vi "Scan.vi"() -> ()   [LabVIEW 2017, in "HP4192A IA.lvclass"]
uses:
  HP4192A IA.lvclass
  Global/GPIB Numbers.vi
  <vilib>/Utility/file.llb/Write To Spreadsheet File (DBL).vi
  File IO/File IO.lvclass
panel:
  in  "Number of Averages":u16 max=20 step=1
  in  "Averaging?":bool
  in  "Frequencies":string
  out "Measurements vs. Frequency":cluster{"Y":dbl[], "Y":dbl[]}[](graph)=[{"Y"=[5.0, 5.0, 5.0, 5.0, 5.0], "Y"=[-246999.99999999997, -1063000.0, -361000.0, -401000.0, -539000.0]}]
  in  "Delay between\nsteps":u32=500
  in  "?":bool
  in  "Append?":bool
  out "Current Frequency":dbl
  in  "?":bool
  in  "L":bool
  in  "C":bool
  in  "R":bool
  in  "Z":bool
  in  "Output File":path=path "C:/Data/Dielectric Measurements/2013 Measurements/.csv"
  # "Measure"
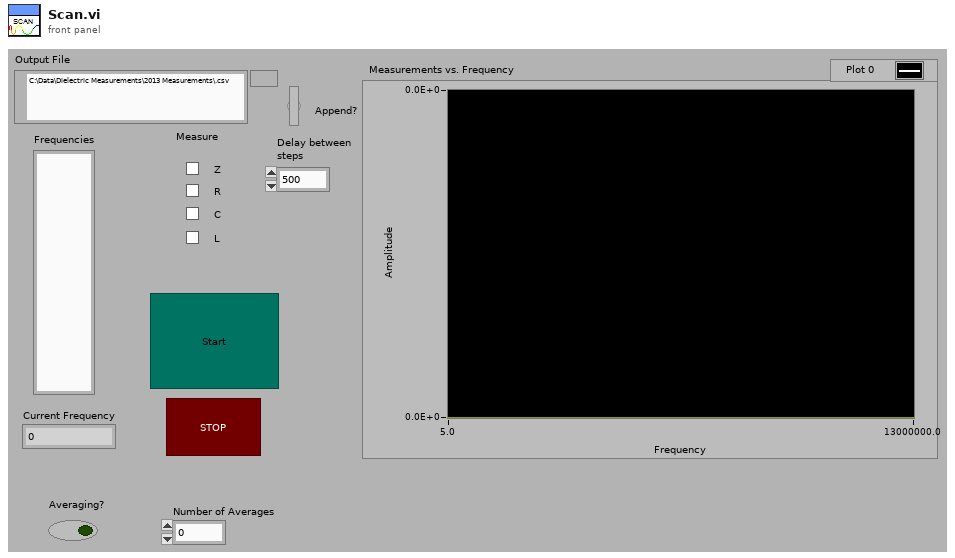
[diagram p1: front panel]
types:
  T1 = typedef "GPIB Type Def.ctl" = cluster{"Name":string, "bus":dbl, "GPIB":dbl, "GPIB as string":string, "byte":i32, "VISA Resource Name":refnum<visa-resource-name>}
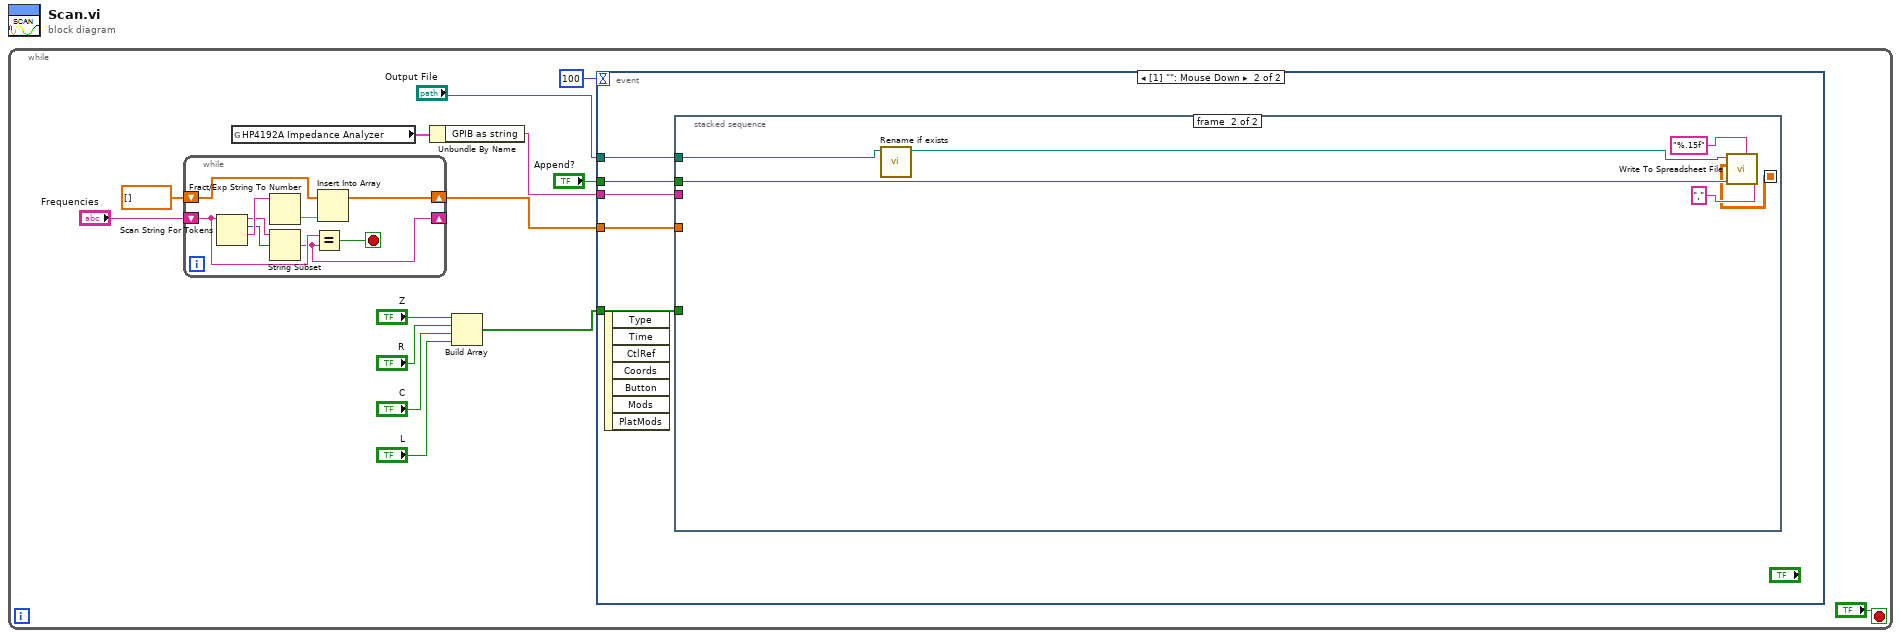
[diagram p0: block diagram]
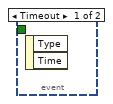
[diagram p2: hidden frame]
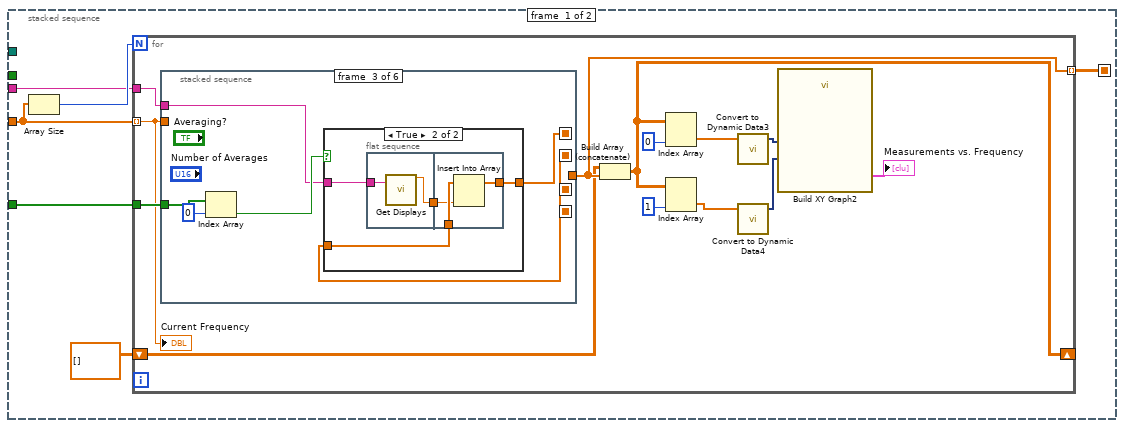
[diagram p3: hidden frame]
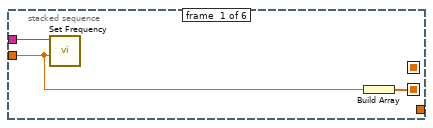
[diagram p4: hidden frame]
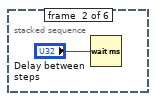
[diagram p5: hidden frame]
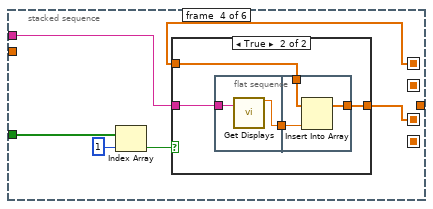
[diagram p7: hidden frame]
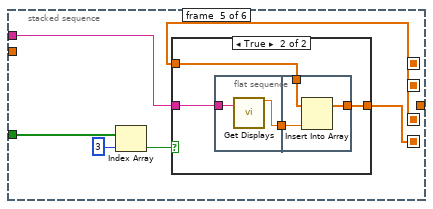
[diagram p9: hidden frame]
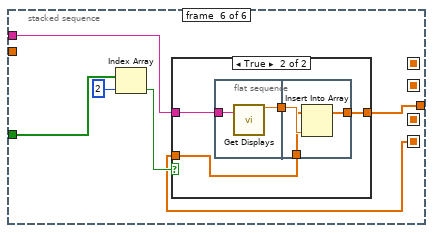
[diagram p11: hidden frame]
diagram:
  n1 = while {
    stop <- "?" stop-if-true
    n2 = while {
      shift-right: [w20] -> w2
      shift-left: dbl[] [] -> [w22]
      shift-right: [w15] -> _
      shift-left: "Frequencies" -> [w18]
      stop <- w17 stop-if-true
      n3 = Scan String For Tokens(9:w18) -> (1:w23:string, 2:w16:i32, 3:w19:string)  [unwired: 5 in, 1 out]
      n4 = Fract/Exp String To Number(string=w23) -> (number=w21:dbl)  [unwired: 3 in, 1 out]
      n5 = String Subset(string=w19, offset (0)=w16) -> (substring=w15:string)  [unwired: 1 in]
      n6 = Equal?(x=w18, y=w15) -> (x = y?=w17:bool)
      n7 = Insert Into Array(array=w22, new element=w21) -> (w20:dbl[])  [unwired: 1 in]
    }
    n8 = global read "GPIB Numbers.vi" "HP4192A Impedance Analyzer"() -> (w7:T1)
    n9 = Unbundle By Name(w7) -> ("GPIB as string"=w6:string)
    n10 = Build Array("Z", "R", "C", "L") -> (w8:bool[])
    n11 = event shown="[1] \"\": Mouse Down" {
      selector: _ -> [_ _]
      dyn-events: _ -> [_ _]
      timeout: 100 -> [_ _]
      tunnel: "Output File" -> [_ w28]
      tunnel: "Append?" -> [_ w27]
      tunnel: w2 -> [_ w26]
      tunnel: w8 -> [_ w25]
      tunnel: w6 -> [_ w24]
      event Timeout {
        n12 = event-data() -> ()  [unwired: 1 in, 2 out]
      }
      event Mouse Down {
        n13 = event-data() -> ()  [unwired: 1 in, 7 out]
        n14 = stacked-sequence {
          seq-local: [w30 _] -> [_ w119]
          tunnel: w28 -> [_ w117]
          tunnel: w27 -> [_ w121]
          tunnel: w26 -> [w33 _]
          tunnel: w25 -> [w32 _]
          tunnel: w24 -> [w31 _]
          frame #0 {
            n15 = Array Size(array=w33) -> (size(s)=w34:i32)
            n16 = for {
              N: w34 -> [_]
              tunnel: w33 -> [w45] mode=indexing
              tunnel: w32 -> [w47]
              tunnel: w31 -> [w46]
              tunnel: [w41] -> w30 mode=indexing
              shift-right: [w39] -> _
              shift-left: dbl[][] [] -> [w40]
              n17 = stacked-sequence {
                seq-local: [w48 _ _ _ _ _] -> [_ _ w54 _ _ _]
                seq-local: [_ _ w52 _ _ _] -> [_ _ _ w69 _ _]
                seq-local: [_ _ _ w68 _ _] -> [_ _ _ _ w88 _]
                seq-local: [_ _ _ _ w84 _] -> [_ _ _ _ _ w101]
                tunnel: w47 -> [_ _ w57 w72 w86 w103]
                tunnel: w46 -> [w50 _ w53 w70 w87 w102]
                tunnel: w45 -> [w49 _ _ _ _ _]
                tunnel: [_ _ _ _ _ w100] -> w41
                frame #0 {
                  n18 = call "Set Frequency.vi"("test signal\nfreq (Hz)"=w49, "GPIB addess"=w50) -> ()  [unwired: 10 in]
                  n19 = Build Array(w49) -> (w48:dbl[])
                }
                frame #1 {
                  n20 = Wait (ms)(milliseconds to wait="Delay between\nsteps") -> ()  [unwired: 1 out]
                }
                frame #2 {
                  n21 = Index Array(array=w57, index=0) -> (element=w55:bool)
                  n22 = case shown="True" w55 {
                    tunnel: w54 -> [w58 w60]
                    tunnel: w53 -> [_ w62]
                    tunnel: [w58 w59] -> w52
                    frame False {
                    }
                    frame True {
                      n23 = flat-sequence {
                        tunnel: w62 -> [w64]
                        tunnel: [w63] -> w61
                        tunnel: w61 -> [w66]
                        tunnel: w60 -> [w67]
                        tunnel: [w65] -> w59
                        frame #0 {
                          n24 = call "Get Displays.vi"("GPIB addess"=w64) -> ("display A"=w63:dbl)  [unwired: 11 in, 7 out]
                        }
                        frame #1 {
                          n25 = Insert Into Array(array=w67, new element=w66) -> (w65:dbl[])  [unwired: 1 in]
                        }
                      }
                    }
                  }
                }
                frame #3 {
                  n26 = Index Array(array=w72, index=1) -> (element=w71:bool)
                  n27 = case shown="True" w71 {
                    tunnel: w70 -> [_ w77]
                    tunnel: w69 -> [w74 w76]
                    tunnel: [w74 w75] -> w68
                    frame False {
                    }
                    frame True {
                      n28 = flat-sequence {
                        tunnel: [w80] -> w78
                        tunnel: w77 -> [w79]
                        tunnel: w78 -> [w83]
                        tunnel: w76 -> [w82]
                        tunnel: [w81] -> w75
                        frame #0 {
                          n29 = call "Get Displays.vi"("GPIB addess"=w79) -> ("display A"=w80:dbl)  [unwired: 11 in, 7 out]
                        }
                        frame #1 {
                          n30 = Insert Into Array(array=w82, new element=w83) -> (w81:dbl[])  [unwired: 1 in]
                        }
                      }
                    }
                  }
                }
                frame #4 {
                  n31 = Index Array(array=w86, index=3) -> (element=w85:bool)
                  n32 = case shown="True" w85 {
                    tunnel: [w90 w93] -> w84
                    tunnel: w88 -> [w90 w92]
                    tunnel: w87 -> [_ w91]
                    frame False {
                    }
                    frame True {
                      n33 = flat-sequence {
                        tunnel: [w96] -> w94
                        tunnel: w91 -> [w95]
                        tunnel: w94 -> [w99]
                        tunnel: [w98] -> w93
                        tunnel: w92 -> [w97]
                        frame #0 {
                          n34 = call "Get Displays.vi"("GPIB addess"=w95) -> ("display A"=w96:dbl)  [unwired: 11 in, 7 out]
                        }
                        frame #1 {
                          n35 = Insert Into Array(array=w97, new element=w99) -> (w98:dbl[])  [unwired: 1 in]
                        }
                      }
                    }
                  }
                }
                frame #5 {
                  n36 = Index Array(array=w103, index=2) -> (element=w104:bool)
                  n37 = case shown="True" w104 {
                    tunnel: [w106 w109] -> w100
                    tunnel: w102 -> [_ w108]
                    tunnel: w101 -> [w106 w107]
                    frame False {
                    }
                    frame True {
                      n38 = flat-sequence {
                        tunnel: [w112] -> w110
                        tunnel: w108 -> [w111]
                        tunnel: w110 -> [w115]
                        tunnel: [w114] -> w109
                        tunnel: w107 -> [w113]
                        frame #0 {
                          n39 = call "Get Displays.vi"("GPIB addess"=w111) -> ("display A"=w112:dbl)  [unwired: 11 in, 7 out]
                        }
                        frame #1 {
                          n40 = Insert Into Array(array=w113, new element=w115) -> (w114:dbl[])  [unwired: 1 in]
                        }
                      }
                    }
                  }
                }
              }
              n41 = Build Array (concatenate)(w40, w41) -> (w39:dbl[][])
              n42 = Index Array(array=w39, index (col)=0) -> (element=w36:dbl[])  [unwired: 1 in]
              n43 = Index Array(array=w39, index (col)=1) -> (element=w35:dbl[])  [unwired: 1 in]
              n44 = call "Convert to Dynamic Data3"("Array"=w36) -> ("Dynamic Data Type"=w37:dynamicdata)  [unwired: 3 in]
              n45 = call "Convert to Dynamic Data4"("Array"=w35) -> ("Dynamic Data Type"=w38:dynamicdata)  [unwired: 3 in]
              n46 = call "Build XY Graph2"("Y Input"=w38, "X Input"=w37) -> ("XY Graph"=→"Measurements vs. Frequency":cluster{"Y":dbl[], "Y":dbl[]}[])  [unwired: 8 in, 1 out]
              "Current Frequency" <- w45
            }
          }
          frame #1 {
            n47 = call "Rename if exists.vi"("File Path"=w117) -> ("New path"=w116:path)  [unwired: 2 in, 8 out]
            n48 = call-poly <vilib>:"Write To Spreadsheet File.vi"("delimiter (\\t)"=",", "format (%.3f)"="%.15f", "append to file? (new file:F)"=w121, "2D data"=w119, "file path (dialog if empty)"=w116) -> ()  [unwired: 3 in, 1 out]
          }
        }
      }
    }
  }
